vi "AddProjectConditionalDeactivationValueByKey.vi"(8 "Fehler (Eingang, kein Fehler)":errorcluster, 10 "CondDeact":cluster{"Keys":string[], "Values":string[]}, 11 "Set":cluster{"Key":string, "Value":string}) -> (0 "Fehler (Ausgang)":errorcluster, 2 "Ausgangs-Cluster":cluster{string[], string[]})   [LabVIEW 2015, in "ConditionalDeactivation.lvlib"]
uses:
  ConditionalDeactivation.lvlib
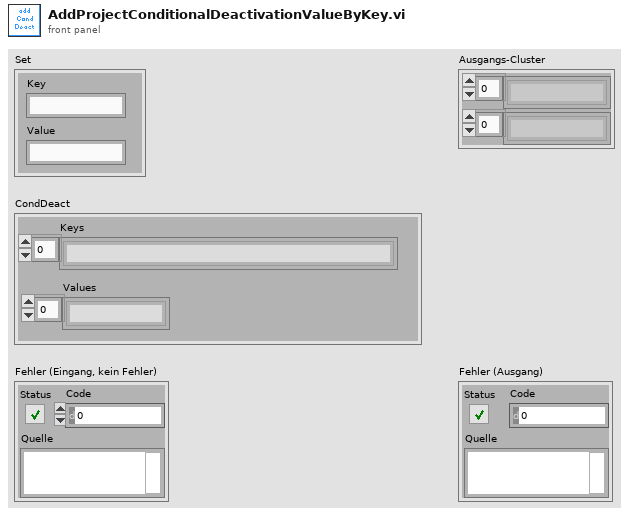
[diagram p1: front panel]
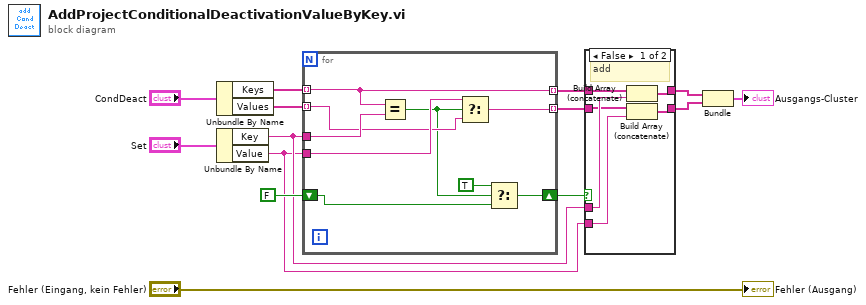
[diagram p0: block diagram]
diagram:
  n1 = Unbundle By Name("CondDeact") -> ("Keys"=w12:string[], "Values"=w11:string[])
  n2 = Unbundle By Name("Set") -> ("Key"=w7:string, "Value"=w6:string)
  n3 = for {
    tunnel: w12 -> [w16] mode=indexing
    tunnel: w11 -> [w21] mode=indexing
    tunnel: w7 -> [w23]
    tunnel: w6 -> [w22]
    shift-right: [w17] -> w8
    shift-left: FALSE -> [w19]
    tunnel: [w16] -> w5 mode=indexing
    tunnel: [w15] -> w4 mode=indexing
    n4 = Equal?(x=w16, y=w23) -> (x = y?=w20:bool)
    n5 = Select(t=w22, s=w20, f=w21) -> (s? t:f=w15:string)
    n6 = Select(t=TRUE, s=w20, f=w19) -> (s? t:f=w17:bool)
  }
  n7 = case shown="False" w8 {
    tunnel: w7 -> [w27 _]
    tunnel: w6 -> [w24 _]
    tunnel: w5 -> [w29 w31]
    tunnel: w4 -> [w26 w30]
    tunnel: [w28 w31] -> w3
    tunnel: [w25 w30] -> w2
    frame False {
      # "add"
      n8 = Build Array (concatenate)(w29, w27) -> (w28:string[])
      n9 = Build Array (concatenate)(w26, w24) -> (w25:string[])
    }
    frame True {
      # "set"
    }
  }
  n10 = Bundle(w3, w2) -> (→"Ausgangs-Cluster":cluster{string[], string[]})  [unwired: 1 in]
  "Fehler (Ausgang)" <- "Fehler (Eingang, kein Fehler)"
